vi "Setup.vi"(11 "Queue Transport in":refnum<class "Queue Transport.lvclass">) -> (0 "Error out":errorcluster, 3 "Queue Transport out":refnum<class "Queue Transport.lvclass">)   [LabVIEW 2025, in "jettl.lvlib" / "Transport.lvlib" / "Queue.lvlib" / "Queue Transport.lvclass"]
uses:
  Queue Transport.lvclass
  Msg/Msg.lvclass
  Queue Transport.lvclass/Queue Transport.ctl
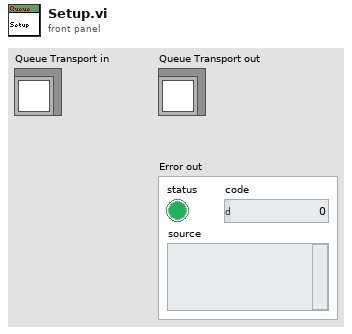
[diagram p1: front panel]
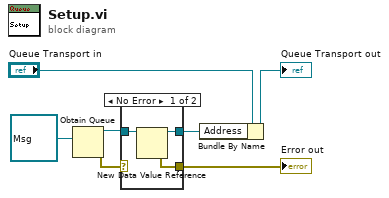
[diagram p0: block diagram]
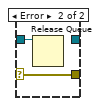
[diagram p2: hidden frame]
diagram:
  n1 = Obtain Queue(element data type=refnum<class "Msg.lvclass"> refnum ("Msg")) -> (queue out=w2:refnum<queue>, error out=w4:errorcluster)  [unwired: 4 in, 1 out]
  n2 = case shown="No Error" w4 {
    selector: w4 -> [_ w12]
    tunnel: [w10 w12] -> w3
    tunnel: w2 -> [w9 w11]
    tunnel: [w8 _] -> w1
    frame No Error {
      n3 = New Data Value Reference(data value=w9) -> (data value reference=w8:refnum<data-value>, error out=w10:errorcluster)  [unwired: 1 in]
    }
    frame Error {
      n4 = Release Queue(queue=w11) -> ()  [unwired: 2 in, 3 out]
    }
  }
  "Error out" <- w3
  n5 = Bundle By Name(cluster="Queue Transport in", "Address"=w1) -> (→"Queue Transport out":refnum<class "Queue Transport.lvclass">)
